vi "Default Instrument Setup.vi"(8 "error in (no error)":errorcluster, 11 "VISA resource name":refnum<visa-resource-name>) -> (0 "error out":errorcluster, 3 "VISA resource name out":refnum<visa-resource-name>)   [LabVIEW 2010, in "Tegam4040.lvlib"]
doc: "This Utility VI sends a default command string to the instrument whenever a new VISA session is opened, or the instrument is reset. \n\nResets:\nOffset 140 (DAC) to 7FFF as required\nOffset 100 ot all opens."
uses:
  Tegam4040.lvlib
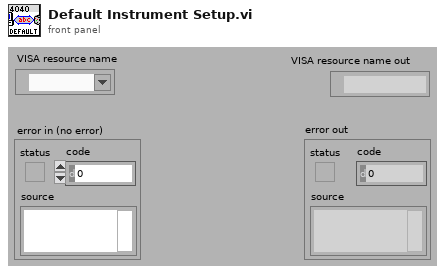
[diagram p1: front panel]
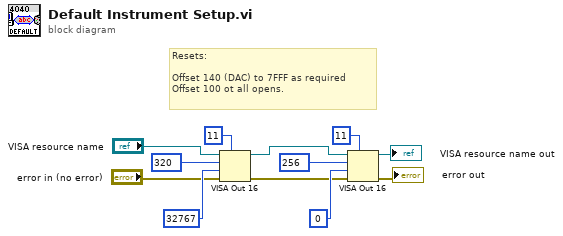
[diagram p0: block diagram]
diagram:
  # "Resets:\n\nOffset 140 (DAC) to 7FFF as required\nOffset 100 ot all opens."
  n1 = VISA Out 16(7:u16 11 ("address space (A16:  1)"), 8:"error in (no error)", 9:u16 32767 ("value (0)"), 10:u32 320 ("offset (0)"), 11:"VISA resource name") -> (0:w3:errorcluster, 3:w4:refnum<visa-resource-name>)
  n2 = VISA Out 16(7:u16 11 ("address space (A16:  1)"), 8:w3, 9:u16 0 ("value (0)"), 10:u32 256 ("offset (0)"), 11:w4) -> (0:→"error out":errorcluster, 3:→"VISA resource name out":refnum<visa-resource-name>)
